vi "IMUMain (1).vi"(8 "error in":errorcluster, 11 "VISA Refnum out":refnum<visa-resource-name>) -> (0 "error out":errorcluster)   [LabVIEW 2017]
doc: "VI dedicated to reading and processing incoming data from IMU (SBG Ellipse)."
uses:
  Sensors/IMUIndex.ctl
  LoopPeriodGLOBAL.vi
  RTControl/StopGLOBAL.vi
panel:
  out "buffer length":i32
  out "msg_id":string
  # "."
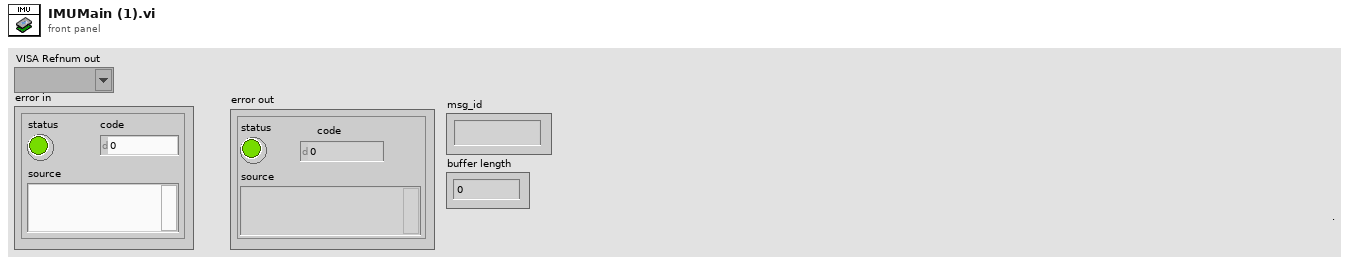
[diagram p1: front panel]
types:
  T1 = typedef "IMUIndex.ctl" = enum16{"Acceleration", "Pressure", "Temperature"}
  T2 = cluster{"TIME_STAMP":u32, "IMU_STATUS":u16, "TEMP":sgl}
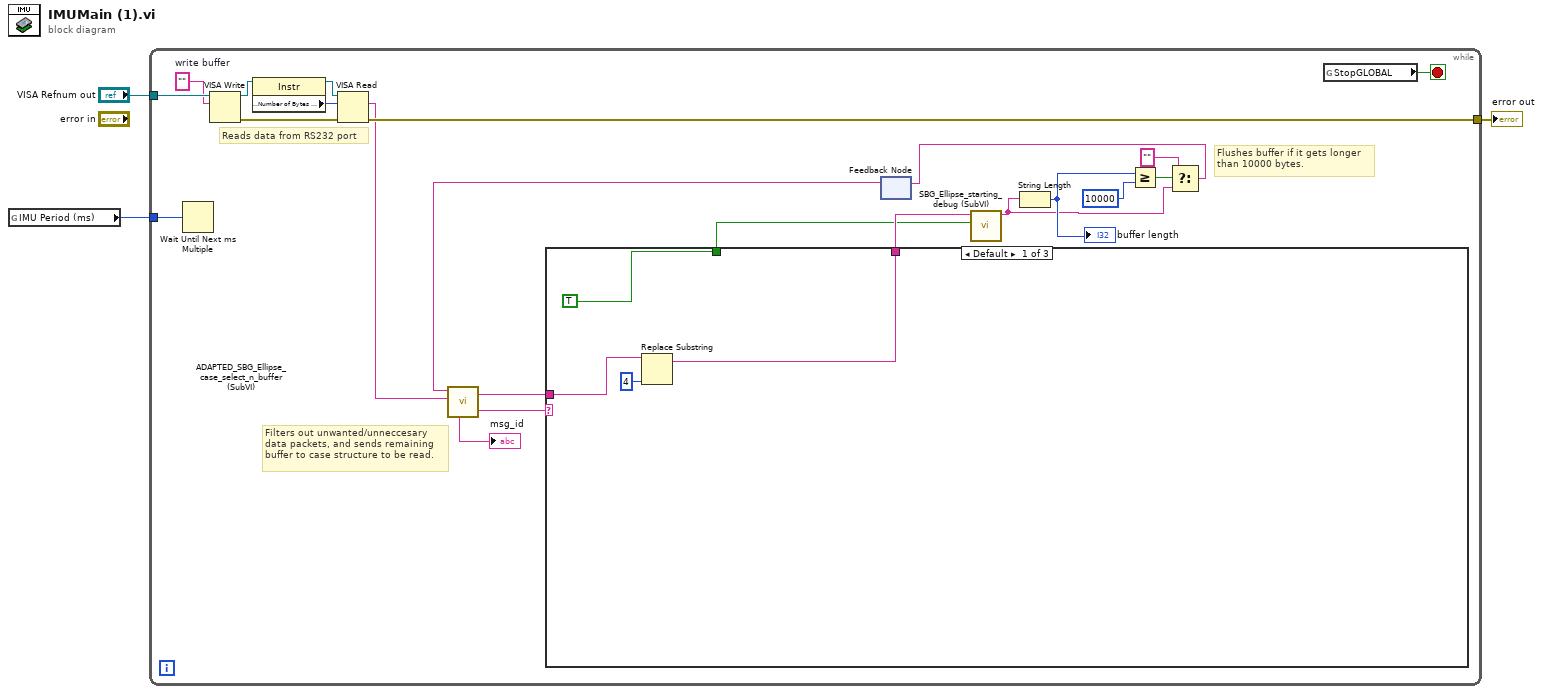
[diagram p0: block diagram]
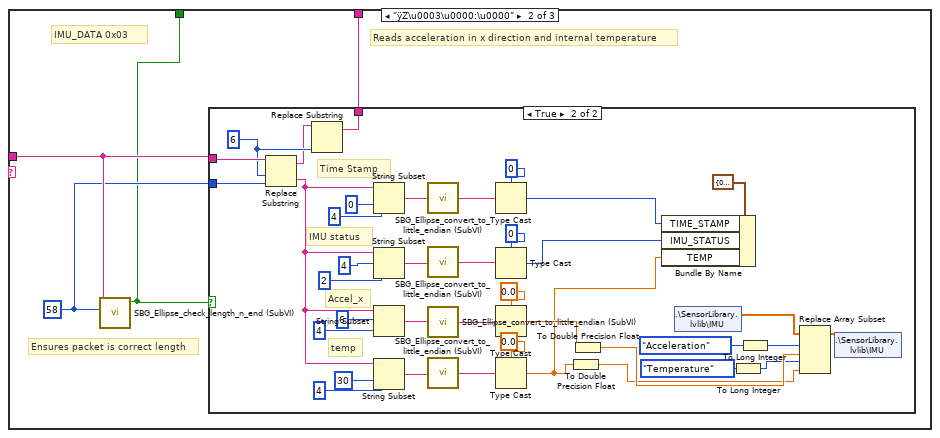
[diagram p2: hidden frame]
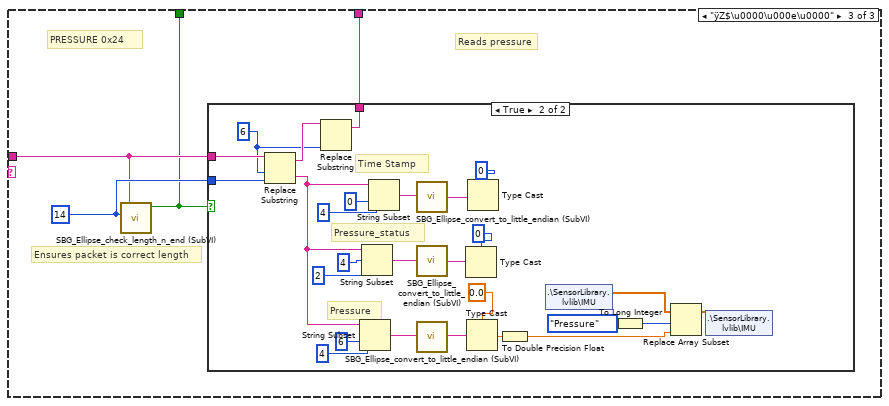
[diagram p4: hidden frame]
diagram:
  n1 = global read "LoopPeriodGLOBAL.vi" "IMU Period (ms)"() -> (w1:u32)
  n2 = while {
    tunnel: "VISA Refnum out" -> [w25]
    tunnel: [w17] -> w2
    tunnel: w1 -> [w5]
    stop <- w4 stop-if-true
    w18 = ""  # write buffer
    # "Filters out unwanted/unneccesary \ndata packets, and sends remaining\nbuffer to case structure to be read."
    # "Reads data from RS232 port"
    # "Flushes buffer if it gets longer\nthan 10000 bytes."
    n3 = Wait Until Next ms Multiple(millisecond multiple=w5) -> ()  [unwired: 1 out]
    n4 = VISA Write(VISA resource name=w25, write buffer=w18) -> (VISA resource name out=w21:refnum<visa-resource-name>, error out=w24:errorcluster)  [unwired: 1 in, 1 out]
    n5 = property class="Instr"(reference=w21) -> (reference out=w22:refnum<visa-resource-name>, "Serial Settings:Number of Bytes at Serial Port"=w23:u32)  [unwired: 1 in, 1 out]
    n6 = VISA Read(VISA resource name=w22, byte count=w23, error in (no error)=w24) -> (read buffer=w15:string, error out=w17:errorcluster)  [unwired: 2 out]
    n7 = feedback #1() -> (w16:string)  [unwired: 1 in]
    n8 = call "ADAPTED_SBG_Ellipse_case_select_n_buffer (SubVI).vi"("new data in"=w15, "buffer data in"=w16) -> ("case_selector"=w13:string, "data out"=w14:string, "msg_id"=→"msg_id":string)  [unwired: 3 in]
    n9 = case shown="Default" w13 {
      tunnel: w14 -> [w28 w32 w76]
      tunnel: [w27 w33 w75] -> w20
      tunnel: [TRUE ("Boolean") w30 w74] -> w19
      frame Default {
        n10 = Replace Substring(2:4 ("length (len. of substring)"), 5:w28) -> (1:w27:string)  [unwired: 2 in, 1 out]
      }
      frame "ÿZ\u0003\u0000:\u0000" {
        w31 = 58 ("x")
        # "Ensures packet is correct length"
        # "Reads acceleration in x direction and internal temperature"
        # "IMU_DATA 0x03"
        n11 = call "SBG_Ellipse_check_length_n_end (SubVI).vi"("x"=w31, "input String"=w32) -> ("is data ok?"=w30:bool)  [unwired: 7 in, 2 out]
        n12 = case shown="True" w30 {
          tunnel: w32 -> [w34 w73]
          tunnel: [w34 w55] -> w33
          tunnel: w31 -> [_ w64]
          frame False {
          }
          frame True {
            w54 = 6 ("length (len. of substring)")
            # "temp"
            # "Accel_x"
            # "IMU status"
            # "Time Stamp"
            n13 = Replace Substring(2:w64, 3:w54, 5:w73) -> (0:w63:string, 1:w53:string)  [unwired: 1 in]
            n14 = Replace Substring(2:w54, 5:w53) -> (1:w55:string)  [unwired: 2 in, 1 out]
            n15 = String Subset(string=w63, offset (0)=0 ("length (len. of substring)"), length (rest)=4 ("length (len. of substring)")) -> (substring=w48:string)
            n16 = String Subset(string=w63, offset (0)=4 ("length (len. of substring)"), length (rest)=2 ("length (len. of substring)")) -> (substring=w47:string)
            n17 = String Subset(string=w63, offset (0)=6 ("length (len. of substring)"), length (rest)=4 ("length (len. of substring)")) -> (substring=w52:string)
            n18 = String Subset(string=w63, offset (0)=30 ("length (len. of substring)"), length (rest)=4 ("length (len. of substring)")) -> (substring=w50:string)
            n19 = call "SBG_Ellipse_convert_to_little_endian (SubVI).vi"("string"=w48) -> ("String"=w45:string)  [unwired: 4 in]
            n20 = call "SBG_Ellipse_convert_to_little_endian (SubVI).vi"("string"=w47) -> ("String"=w46:string)  [unwired: 4 in]
            n21 = call "SBG_Ellipse_convert_to_little_endian (SubVI).vi"("string"=w52) -> ("String"=w51:string)  [unwired: 4 in]
            n22 = call "SBG_Ellipse_convert_to_little_endian (SubVI).vi"("string"=w50) -> ("String"=w49:string)  [unwired: 4 in]
            n23 = Type Cast(type=u32 0, x=w45) -> (*(type *) &x=w57:u32)
            n24 = Type Cast(type=u16 0, x=w46) -> (*(type *) &x=w56:u16)
            n25 = Type Cast(type=sgl 0.0, x=w51) -> (*(type *) &x=w44:sgl)
            n26 = Type Cast(type=sgl 0.0, x=w49) -> (*(type *) &x=w43:sgl)
            n27 = To Double Precision Float(number=w43) -> (double precision float=w39:dbl)
            n28 = To Double Precision Float(number=w44) -> (double precision float=w40:dbl)
            n29 = Bundle By Name(cluster=T2 {"TIME_STAMP"=0, "IMU_STATUS"=0, "TEMP"=0.0}, "TIME_STAMP"=w57, "IMU_STATUS"=w56, "TEMP"=w43) -> ()  [unwired: 1 out]
            n30 = shared-variable ".\\SensorLibrary.lvlib\\IMU"() -> (w41:dbl[])  [unwired: 1 in, 1 out]
            n31 = To Long Integer(number=IMUIndex."Temperature" ("IMU Index")) -> (32bit integer=w35:i32)
            n32 = To Long Integer(number=IMUIndex."Acceleration" ("IMU Index")) -> (32bit integer=w36:i32)
            n33 = Replace Array Subset(array=w41, new element #1=w40, index #1=w36, new element #2=w39, index #2=w35) -> (w42:dbl[])
            n34 = shared-variable ".\\SensorLibrary.lvlib\\IMU"(w42) -> ()  [unwired: 1 in, 1 out]
          }
        }
      }
      frame "ÿZ$\u0000\u000e\u0000" {
        w77 = 14 ("x")
        # "Reads pressure"
        # "Ensures packet is correct length"
        # "PRESSURE 0x24"
        n35 = call "SBG_Ellipse_check_length_n_end (SubVI).vi"("x"=w77, "input String"=w76) -> ("is data ok?"=w74:bool)  [unwired: 7 in, 2 out]
        n36 = case shown="True" w74 {
          tunnel: w76 -> [w78 w105]
          tunnel: [w78 w91] -> w75
          tunnel: w77 -> [_ w98]
          frame False {
          }
          frame True {
            w92 = 6 ("length (len. of substring)")
            # "Pressure"
            # "Pressure_status"
            # "Time Stamp"
            n37 = Replace Substring(2:w98, 3:w92, 5:w105) -> (0:w97:string, 1:w93:string)  [unwired: 1 in]
            n38 = Replace Substring(2:w92, 5:w93) -> (1:w91:string)  [unwired: 2 in, 1 out]
            n39 = String Subset(string=w97, offset (0)=6 ("length (len. of substring)"), length (rest)=4 ("length (len. of substring)")) -> (substring=w86:string)
            n40 = String Subset(string=w97, offset (0)=4 ("length (len. of substring)"), length (rest)=2 ("length (len. of substring)")) -> (substring=w88:string)
            n41 = String Subset(string=w97, offset (0)=0 ("length (len. of substring)"), length (rest)=4 ("length (len. of substring)")) -> (substring=w90:string)
            n42 = call "SBG_Ellipse_convert_to_little_endian (SubVI).vi"("string"=w90) -> ("String"=w89:string)  [unwired: 4 in]
            n43 = call "SBG_Ellipse_convert_to_little_endian (SubVI).vi"("string"=w88) -> ("String"=w87:string)  [unwired: 4 in]
            n44 = call "SBG_Ellipse_convert_to_little_endian (SubVI).vi"("string"=w86) -> ("String"=w85:string)  [unwired: 4 in]
            n45 = Type Cast(type=u16 0, x=w87) -> ()  [unwired: 1 out]
            n46 = Type Cast(type=sgl 0.0, x=w85) -> (*(type *) &x=w84:sgl)
            n47 = Type Cast(type=u32 0, x=w89) -> ()  [unwired: 1 out]
            n48 = To Double Precision Float(number=w84) -> (double precision float=w81:dbl)
            n49 = shared-variable ".\\SensorLibrary.lvlib\\IMU"() -> (w83:dbl[])  [unwired: 1 in, 1 out]
            n50 = To Long Integer(number=IMUIndex."Pressure" ("IMU Index")) -> (32bit integer=w79:i32)
            n51 = Replace Array Subset(array=w83, new element=w81, index=w79) -> (w82:dbl[])
            n52 = shared-variable ".\\SensorLibrary.lvlib\\IMU"(w82) -> ()  [unwired: 1 in, 1 out]
          }
        }
      }
    }
    n53 = call "SBG_Ellipse_starting_debug (SubVI).vi"("boolean from check"=w19, "result string in"=w20) -> ("result string out"=w8:string)  [unwired: 9 in]
    n54 = String Length(string=w8) -> (length=w11:i32)
    "buffer length" <- w11
    n55 = Greater Or Equal?(x=w11, y=10000) -> (x >= y?=w9:bool)
    n56 = Select(t="", s=w9, f=w8) -> (s? t:f=w6:string)
    n57 = feedback-in #1(w6) -> ()
    n58 = global read "StopGLOBAL.vi" "StopGLOBAL"() -> (w4:bool)
  }
  "error out" <- w2
